vi "Determine Playable.vi"(11 "Status":T1={"VI"={"error"={"status"=FALSE, "code"=0, "source"=""}, "isExiting?"=FALSE}, "UserLoggedIn?"=FALSE, "Processors"={"Averaging Type"=enum."Normal Average", "Roughness Processor"=refnum, "Objects"={"Video A"=refnum, "Video B"=refnum}}, "Playback"={"FPS"=10.0, "Playing?"=FALSE, "Playable?"=FALSE, "Image A"=refnum, "Image B"=refnum}, "Mouse Position A"=0.0, "Mouse Position B"=0.0, "Camera Settings"={"Use Camera A?"=FALSE, "Use Camera B?"=FALSE, "Device Index A"=0, "Device Index B"=0, "Sensor Index A"=0, "Sensor Index B"=0}}) -> (3 "Status Out":T1={"VI"={"error"={"status"=FALSE, "code"=0, "source"=""}, "isExiting?"=FALSE}, "UserLoggedIn?"=FALSE, "Processors"={"Averaging Type"=enum."Normal Average", "Roughness Processor"=refnum, "Objects"={"Video A"=refnum, "Video B"=refnum}}, "Playback"={"FPS"=10.0, "Playing?"=FALSE, "Playable?"=FALSE, "Image A"=refnum, "Image B"=refnum}, "Mouse Position A"=0.0, "Mouse Position B"=0.0, "Camera Settings"={"Use Camera A?"=FALSE, "Use Camera B?"=FALSE, "Device Index A"=0, "Device Index B"=0, "Sensor Index A"=0, "Sensor Index B"=0}})   [LabVIEW 2018]
uses:
  Status STYP.ctl
  Roughness Averager/Roughness Averager.lvclass
  Video File/Video File.lvclass
  <vilib>/vision/Image Controls.llb/IMAQ Image.ctl
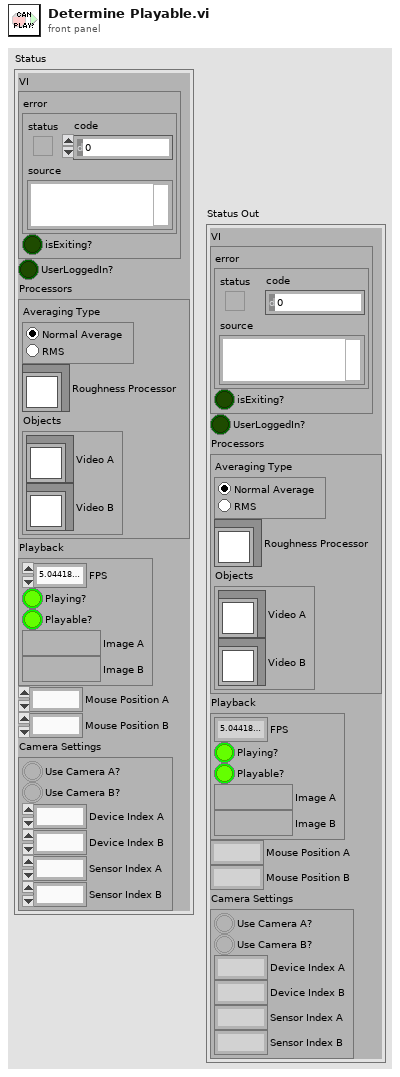
[diagram p1: front panel]
types:
  T1 = typedef "Status STYP.ctl" = cluster{"VI":cluster{"error":errorcluster, "isExiting?":bool}, "UserLoggedIn?":bool, "Processors":cluster{"Averaging Type":enum32{"Normal Average", "RMS"}, "Roughness Processor":refnum<class "Roughness Averager.lvclass">, "Objects":cluster{"Video A":refnum<class "Video File.lvclass">, "Video B":refnum<class "Video File.lvclass">}}, "Playback":cluster{"FPS":dbl, "Playing?":bool, "Playable?":bool, "Image A":T2, "Image B":T2}, "Mouse Position A":dbl, "Mouse Position B":dbl, "Camera Settings":cluster{"Use Camera A?":bool, "Use Camera B?":bool, "Device Index A":i32, "Device Index B":i32, "Sensor Index A":i32, "Sensor Index B":i32}}
  T2 = typedef "IMAQ Image.ctl" = refnum<image>
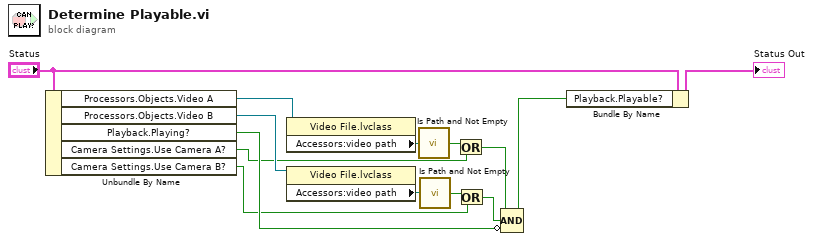
[diagram p0: block diagram]
diagram:
  n1 = Unbundle By Name("Status") -> ("Processors.Objects.Video A"=w14:refnum<class "Video File.lvclass">, "Processors.Objects.Video B"=w13:refnum<class "Video File.lvclass">, "Playback.Playing?"=w8:bool, "Camera Settings.Use Camera A?"=w2:bool, "Camera Settings.Use Camera B?"=w1:bool)
  n2 = property class="Video File.lvclass"(reference=w14) -> ("Accessors:video path"=w12:path)  [unwired: 1 in, 2 out]
  n3 = property class="Video File.lvclass"(reference=w13) -> ("Accessors:video path"=w11:path)  [unwired: 1 in, 2 out]
  n4 = call <vilib>:"Is Path and Not Empty.vi"("path"=w12) -> ("Is Path and Not Empty?"=w10:bool)  [unwired: 4 in]
  n5 = call <vilib>:"Is Path and Not Empty.vi"("path"=w11) -> ("Is Path and Not Empty?"=w9:bool)  [unwired: 4 in]
  n6 = Or(x=w10, y=w2) -> (x .or. y?=w4:bool)
  n7 = Or(x=w9, y=w1) -> (x .or. y?=w3:bool)
  n8 = Compound Arithmetic op=AND(w4, w3, invert w8) -> (w6:bool)
  n9 = Bundle By Name(cluster="Status", "Playback.Playable?"=w6) -> (→"Status Out":T1)
